vi "RingBlockSel.VI"() -> ()   [LabVIEW 2014]
panel:
  in  "hi&lo \nslope":bool=TRUE
  in  "DAT in 10ns":u32
  in  "ext block trig example":bool
  in  "stop fetch":bool
  in  "Stopp":bool
  in  "Stop":i32=10
  in  "Start":i32=-10
  in  "select scan":i32(slide) scale=-10.0..10.0
  out "FIFO overflow":bool
  in  "RingBufDepth":u32=25
  out "Signalverlaufgraph":u16[](graph)=[1267, 50417, 4112, 1267, 7659, 7696, 7725, 7725, 7755, 7770, 7795, 7766, 7742, 7841, 7891, 7865, 7946, 7910, 7955, 7940, 7976, 7982, 8030, 8028, 8081, 8037, 8122, 8111, 8154, 8145, 8187, 8182, 8231, 8225, 8281, 8262, 8310, 8296, 8347, 8333, 8376, 8398, 8432, 8403, 8476, 8449, 8510, 8489, 8525, 8545, 8582, 8581, 8618, 8613, 8667, 8654, 8692, 8708, 8759, 8706, 8745, 8782, 8814, 8809, 8848, 8846, 8898, 8851, 8926, 8918, 8947, 8949, 8990, 8954, 8988, 9025, 9062, 9045, 9104, 9090, 9093, 9115, 9157, 9189, 9229, 9158, 9258, 9245, 9271, 9314, 9327, 9359, 9410, 9377, 9420, 9443, 9452, 9480, 9515, 9525, 9564, 9554, 9535, 9526, 9597, 9626, 9693, 9690, 9715, 9722, 9769, 9773, 9771, 9758, 9816, 9815, 9862, 9880, 9862, 9878, 9937, 9924, 9971, 9973, 10030, 10038, 10047, 10060, 10091, 10102, 10098, 10114, 10184, 10164, 10217, 10205, 10257, 10232, 10302, 10288, 10306, 10337, 10390, 10402, 10412, 10450, 10469, 10377, 10424, 10490, 10536, 10563, 10586, 10615, 10624, 10632, 10669, 10670, 10730, 10717, 10761, 10729, 10815, 10842, 10839, 10803, 10887, 10862, 10917, 10908, 10955, 10977, 11004, 11014, 11032, 11051, 11095, 11125, 11146, 11144, 11172, 11218, 11222, 11277, 11288, 11293, 11342, 11330, 11365, 11358, 11468, 11450, 11496, 11467, 11546, 11548, 11575, 11579, 11632, 11635, 11652, 11669, 11737, 11683, 11749, 11767, 11790, 11804, 11845, 11814, 11890, 11779, 11834, 11919, 11972, 11959, 11983, 12001, 12073, 12051, 12097, 12065, 12122, 12126, 12074, 12173, 12211, 12175, 12289, 12285, 12296, 12283, 12293, 12301, 12367, 12362, 12415, 12470, 12439, 12441, 12502, 12486, 12596, 12510, 12601, 12597, 12602, 12572, 12645, 12624, 12735, 12688, 12767, 12739, 12766, 12773, 12767, 12772, 12833, 12801, 12902, 12819, 12890, 12935, 12947, 12911, 12942, 12985, 12965, 12990, 13062, 13021, 12998, 13051, 13106, 13089, 13085, 13126, 13151, 13167, 13155, 13130, 13159, 13244, 13205, 13274, 13270, 13265, 13291, 13315, 13327, 13383, 13278, 13409, 13379, 13376, 13384, 13367, 13442, 13461, 13478, 13463, 13460, 13488, 13475, 13512, 13533, 13544, 13587, 13557, 13565, 13570, 13564, 13619, 13631, 13616, 13606, 13613, 13635, 13670, 13669, 13623, 13680, 13702, 13694, 13688, 13803, 13723, 13749, 13747, 13704, 13670, 13674, 13609, 13710, 13778, 13763, 13750, 13722, 13756, 13688, 13716, 13707, 13769, 13716, 13741, 13764, 13729, 13759, 13799, 13759, 13772, 13784, 13736, 13809, 13711, 13812, 13757, 13736, 13770, 13760, 13730, 13797, 13712, 13746, 13752, 13738, 13686, 13747, 13737, 13749, 13705, 13718, 13759, 13717, 13643, 13689, 13642, 13658, 13682, 13671, 13659, 13670, 13630, 13670, 13604, 13624, 13626, 13612, 13620, 13626, 13612, 13622, 13589, 13626, 13563, 13551, 13541, 13554, 13592, 13534, 13493, 13501, 13521, 13493, 13450, 13478, 13454, 13499, 13456, 13451, 13410, 13442, 13409, 13444, 13420, 13400, 13375, 13402, 13392, 13369, 13360, 13375, 13345, 13378, 13309, 13303, 13341, 13341, 13295, 13312, 13261, 13243, 13305, 13260, 13245, 13230, 13226, 13217, 13219, 13205, 13138, 13201, 13081, 13157, 13137, 13152, 13177, 13116, 13104, 13060, 13100, 13070, 13052, 13019, 13064, 13010, 13015, 12965, 12979, 12970, 12985, 12973, 12950, 12926, 12889, 12864, 12859, 12835, 12861, 12815, 12800, 12763, 12772, 12762, 12743, 12693, 12754, 12692, 12686, 12660, 12656, 12634, 12607, 12590, 12610, 12472, 12565, 12457, 12494, 12477, 12435, 12473, 12428, 12376, 12385, 12323, 12353, 12271, 12306, 12241, 12270, 12196, 12222, 12149, 12184, 12123, 12176, 12105, 12118, 12066, 12062, 11982, 11953, 11919, 11930, 1283, 1294, 1292, 1293, 1298, 1290, 1294, 1294, 1298, 1294, 1295, 1293, 1285, 1284, 1285, 1286, 1281, 1283, 1286, 1284, 1282, 1276, 1283, 1273, 1278, 1276, 1272, 1273, 1275, 1278, 1273, 1273, 1267, 1266]
  in  "Trigger":bool
  in  "ClrReads":u32=4
  in  "exposuretime":dbl=1.0 format="%.2f"
  # "Start with run"
  # "be shure to use lower stop button or ESC to quit - or thread will keep on going!"
  # "in ms"
  # "ext"
  # "int"
  # "timer example"
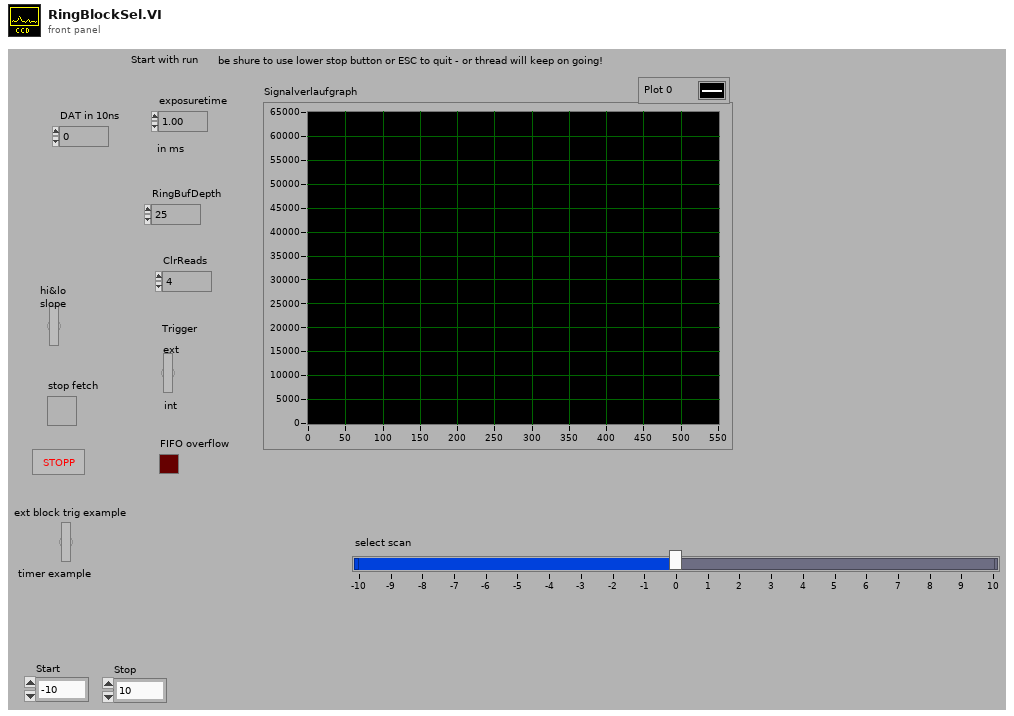
[diagram p1: front panel]
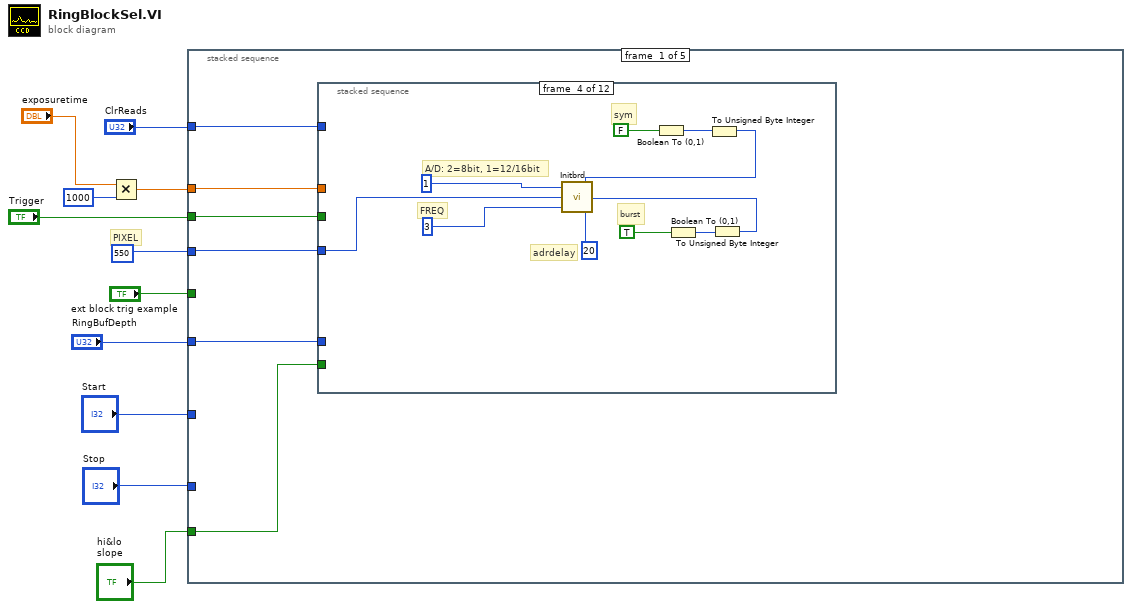
[diagram p0: block diagram]
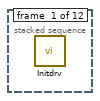
[diagram p2: hidden frame]
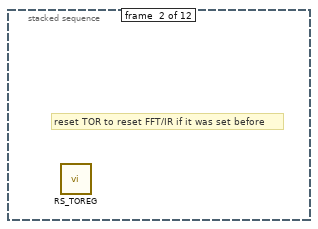
[diagram p3: hidden frame]
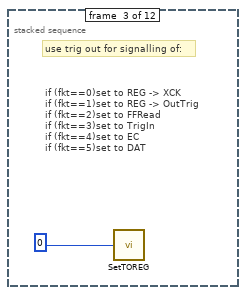
[diagram p4: hidden frame]
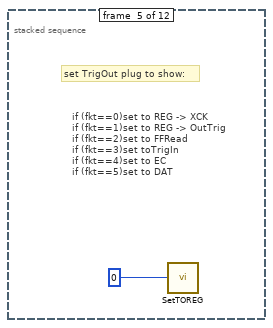
[diagram p5: hidden frame]
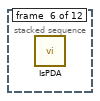
[diagram p6: hidden frame]
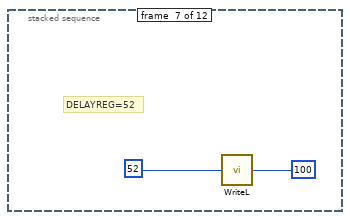
[diagram p7: hidden frame]
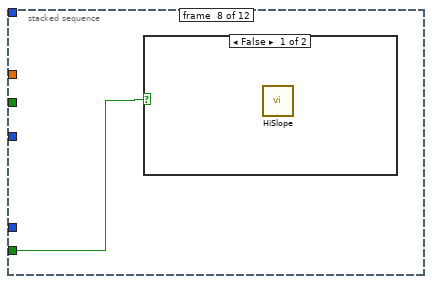
[diagram p8: hidden frame]
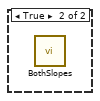
[diagram p9: hidden frame]
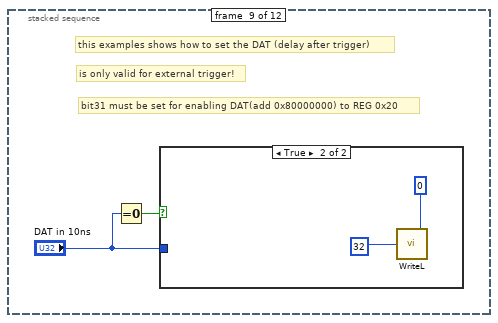
[diagram p10: hidden frame]
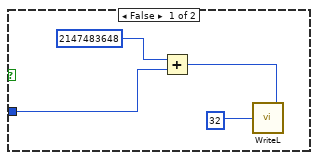
[diagram p11: hidden frame]
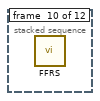
[diagram p12: hidden frame]
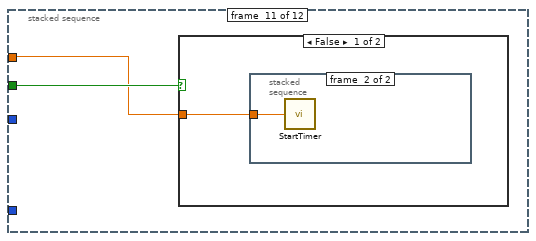
[diagram p13: hidden frame]
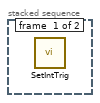
[diagram p14: hidden frame]
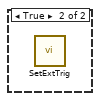
[diagram p15: hidden frame]
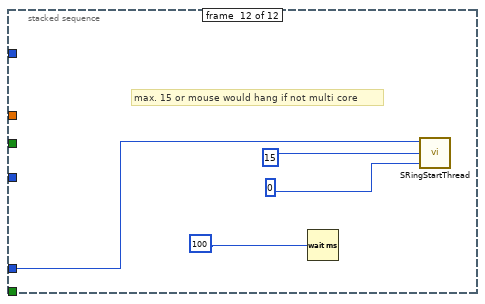
[diagram p16: hidden frame]
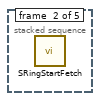
[diagram p17: hidden frame]
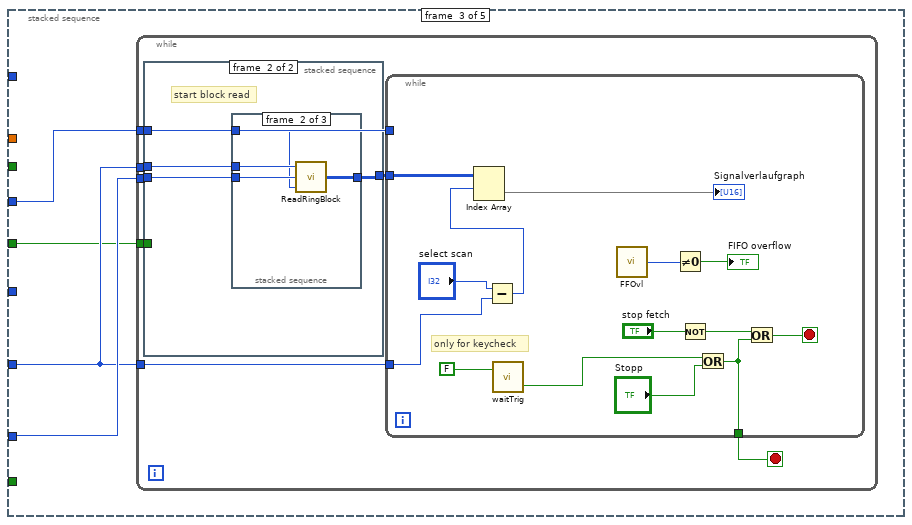
[diagram p18: hidden frame]
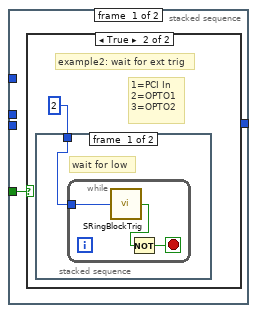
[diagram p19: hidden frame]
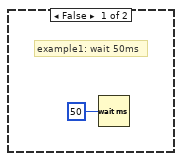
[diagram p20: hidden frame]
diagram:
  # "PIXEL"
  n1 = Multiply(x="exposuretime", y=1000) -> (x*y=w7:dbl)
  n2 = stacked-sequence {
    tunnel: w7 -> [w16 _ _ _ _]
    tunnel: u32 550 -> [w17 _ w52 _ _]
    tunnel: "ClrReads" -> [w15 _ _ _ _]
    tunnel: "Trigger" -> [w14 _ _ _ _]
    tunnel: "RingBufDepth" -> [w13 _ _ _ _]
    tunnel: "Stop" -> [_ _ w51 _ _]
    tunnel: "Start" -> [_ _ w50 _ _]
    tunnel: "ext block trig example" -> [_ _ w49 _ _]
    tunnel: "hi&lo \nslope" -> [w12 _ _ _ _]
    frame #0 {
      n3 = stacked-sequence {
        tunnel: w17 -> [_ _ _ w27 _ _ _ _ _ _ _ _]
        tunnel: w16 -> [_ _ _ _ _ _ _ _ _ _ w41 _]
        tunnel: w15 -> [_ _ _ _ _ _ _ _ _ _ _ _]
        tunnel: w14 -> [_ _ _ _ _ _ _ _ _ _ w42 _]
        tunnel: w13 -> [_ _ _ _ _ _ _ _ _ _ _ w45]
        tunnel: w12 -> [_ _ _ _ _ _ _ w32 _ _ _ _]
        frame #0 {
          n4 = call "Initdrv.vi"() -> ()  [unwired: 1 in]
        }
        frame #1 {
          # "reset TOR to reset FFT/IR if it was set before"
          n5 = call "RS_TOREG.vi"() -> ()  [unwired: 1 in]
        }
        frame #2 {
          # "use trig out for signalling of:"
          # "if (fkt==0)set to REG -> XCK\nif (fkt==1)set to REG -> OutTrig\nif (fkt==2)set to FFRead\nif (fkt==3)set to TrigIn\nif (fkt==4)set to EC\nif (fkt==5)set to DAT"
          n6 = call "SetTOREG.vi"("fkt"=u8 0) -> ()
        }
        frame #3 {
          # "adrdelay"
          # "FREQ"
          # "A/D: 2=8bit, 1=12/16bit"
          # "burst"
          # "sym"
          n7 = Boolean To (0,1)(Boolean=FALSE) -> (0, 1=w21:i16)
          n8 = Boolean To (0,1)(Boolean=TRUE) -> (0, 1=w20:i16)
          n9 = To Unsigned Byte Integer(number=w21) -> (unsigned 8bit integer=w22:u8)
          n10 = To Unsigned Byte Integer(number=w20) -> (unsigned 8bit integer=w19:u8)
          n11 = call "Initbrd.vi"("AdrDelay"=u32 20, "burst"=w19, "sym"=w22, "waits"=u32 3, "pixel"=w27, "flag816"=u32 1) -> ()
        }
        frame #4 {
          # "set TrigOut plug to show:"
          # "if (fkt==0)set to REG -> XCK\nif (fkt==1)set to REG -> OutTrig\nif (fkt==2)set to FFRead\nif (fkt==3)set toTrigIn\nif (fkt==4)set to EC\nif (fkt==5)set to DAT"
          n12 = call "SetTOREG.vi"("fkt"=u8 0) -> ()
        }
        frame #5 {
          n13 = call "IsPDA.vi"() -> ()  [unwired: 1 in]
        }
        frame #6 {
          # "DELAYREG=52"
          n14 = call "WriteL.vi"("val"=u32 100, "offset"=u32 52) -> ()
        }
        frame #7 {
          n15 = case shown="False" w32 {
            frame False {
              n16 = call "HiSlope.vi"() -> ()  [unwired: 1 in]
            }
            frame True {
              n17 = call "BothSlopes.vi"() -> ()  [unwired: 1 in]
            }
          }
        }
        frame #8 {
          # "bit31 must be set for enabling DAT(add 0x80000000) to REG 0x20"
          # "is only valid for external trigger!"
          # "this examples shows how to set the DAT (delay after trigger)"
          n18 = Equal To 0?(x="DAT in 10ns") -> (x = 0?=w33:bool)
          n19 = case shown="True" w33 {
            tunnel: "DAT in 10ns" -> [w35 _]
            frame False {
              n20 = Add(x=u32 2147483648, y=w35) -> (x+y=w38:u32)
              n21 = call "WriteL.vi"("val"=w38, "offset"=u32 32) -> ()
            }
            frame True {
              n22 = call "WriteL.vi"("val"=0, "offset"=u32 32) -> ()
            }
          }
        }
        frame #9 {
          n23 = call "FFRS.VI"() -> ()  [unwired: 1 in]
        }
        frame #10 {
          n24 = case shown="False" w42 {
            tunnel: w41 -> [w43 _]
            frame False {
              n25 = stacked-sequence {
                tunnel: w43 -> [_ w44]
                frame #0 {
                  n26 = call "SetIntTrig.vi"() -> ()  [unwired: 1 in]
                }
                frame #1 {
                  n27 = call "StartTimer.vi"("exposure time"=w44) -> ()  [unwired: 1 in]
                }
              }
            }
            frame True {
              n28 = call "SetExtTrig.vi"() -> ()  [unwired: 1 in]
            }
          }
        }
        frame #11 {
          # "max. 15 or mouse would hang if not multi core"
          n29 = Wait (ms)(milliseconds to wait=u32 100) -> ()  [unwired: 1 out]
          n30 = call "SRingStartThread.vi"("releasems"=i16 0, "threadp"=u32 15, "ringdepth"=w45) -> ()  [unwired: 1 in]
        }
      }
    }
    frame #1 {
      n31 = call "SRingStartFetch.vi"() -> ()  [unwired: 2 in]
    }
    frame #2 {
      n32 = while {
        tunnel: w52 -> [w56]
        tunnel: w51 -> [w58]
        tunnel: w50 -> [w57]
        tunnel: w50 -> [w54]
        tunnel: w49 -> [w53]
        stop <- w55 stop-if-true
        n33 = stacked-sequence {
          tunnel: [_ w73] -> w59
          tunnel: w58 -> [_ w72]
          tunnel: w57 -> [_ w71]
          tunnel: w56 -> [_ w70]
          tunnel: w53 -> [w60 _]
          frame #0 {
            n34 = case shown="True" w60 {
              frame False {
                # "example1: wait 50ms"
                n35 = Wait (ms)(milliseconds to wait=u32 50) -> ()  [unwired: 1 out]
              }
              frame True {
                # "1=PCI In\n2=OPTO1\n3=OPTO2"
                # "example2: wait for ext trig"
                n36 = stacked-sequence {
                  tunnel: u8 2 -> [w63 w67]
                  frame #0 {
                    # "wait for low"
                    n37 = while {
                      tunnel: w63 -> [w64]
                      stop <- w66 stop-if-true
                      n38 = call "SRingBlockTrig.vi"("channel 1, 2 or 3"=w64) -> ("Boolesch"=w65:bool)
                      n39 = Not(x=w65) -> (.not. x?=w66:bool)
                    }
                  }
                  frame #1 {
                    # "wait for high"
                    n40 = while {
                      tunnel: w67 -> [w68]
                      stop <- w69 stop-if-true
                      n41 = call "SRingBlockTrig.vi"("channel 1, 2 or 3"=w68) -> ("Boolesch"=w69:bool)
                    }
                  }
                }
              }
            }
          }
          frame #1 {
            # "start block read"
            n42 = stacked-sequence {
              tunnel: [_ w77 _] -> w73
              tunnel: w72 -> [_ w76 _]
              tunnel: w71 -> [_ w75 _]
              tunnel: w70 -> [_ w74 _]
              frame #0 {
                n43 = call "OTrig_h.vi"() -> ()  [unwired: 1 in]
              }
              frame #1 {
                n44 = call "ReadRingBlock.vi"("pixel"=w74, "stop"=w76, "start"=w75) -> ("Data Values"=w77:u16[][])
              }
              frame #2 {
                n45 = call "OTrig_l.vi"() -> ()  [unwired: 1 in]
              }
            }
          }
        }
        n46 = while {
          tunnel: w59 -> [w79]
          tunnel: w56 -> [_]
          tunnel: [w83] -> w55
          tunnel: w54 -> [w86]
          stop <- w89 stop-if-true
          # "only for keycheck"
          n47 = Subtract(x="select scan", y=w86) -> (x-y=w78:i32)
          n48 = Index Array(array=w79, index (row)=w78) -> (element=→"Signalverlaufgraph":u16[])  [unwired: 1 in]
          n49 = call "waitTrig.vi"("Trigger\nextern"=FALSE) -> ("ESCKey"=w81:bool)  [unwired: 1 in, 1 out]
          n50 = call "FFOvl.vi"() -> ("FFOvl"=w91:u8)  [unwired: 1 in]
          n51 = Not Equal To 0?(x=w91) -> (x != 0?=→"FIFO overflow":bool)
          n52 = Not(x="stop fetch") -> (.not. x?=w85:bool)
          n53 = Or(x=w81, y="Stopp") -> (x .or. y?=w83:bool)
          n54 = Or(x=w85, y=w83) -> (x .or. y?=w89:bool)
        }
      }
    }
    frame #3 {
      # "stop thread and timer"
      n55 = stacked-sequence {
        frame #0 {
          n56 = call "SRingStopThread.vi"() -> ()  [unwired: 4 in]
        }
        frame #1 {
          # "be shure not to exit before thread is stopped!"
          n57 = while {
            stop <- w92 continue-if-true
            n58 = call "SRingThreadIsOFF.vi"() -> ("ThreadIsOFF"=w93:u8)  [unwired: 1 in]
            n59 = Equal To 0?(x=w93) -> (x = 0?=w92:bool)
          }
        }
        frame #2 {
          n60 = call "FFStopTimer.vi"() -> ()  [unwired: 1 in]
        }
        frame #3 {
          # "stops ext trigger from running"
          n61 = call "SetIntTrig.vi"() -> ()  [unwired: 1 in]
        }
      }
    }
    frame #4 {
      n62 = call "Exit.vi"() -> ()  [unwired: 1 in]
    }
  }
